vi "DAQmx.Create Trigger.vi"(8 "error in (no error)":errorcluster, 11 "DAQmx in":refnum<class "DAQmx.lvclass">) -> (0 "error out":errorcluster, 3 "DAQmx out":refnum<class "DAQmx.lvclass">)   [LabVIEW 2019, in "DAQmx.lvclass"]
uses:
  DAQmx.lvclass
  typedefs/DAQ.Config.Device Type--enum.ctl
  DAQmx.lvclass/DAQmx.ctl
  a451efbf-a4cf-4ff4-9d43-e4341e5b5646.vi
  <vilib>/DAQmx/configure/trigger.llb/DAQmx Start Trigger (Digital Edge).vi
  <resource>/objmgr/daqmx.rc
panel:
  out "Inventory":cluster{"DAQ Type":T1, "number":i32}[](array[cluster])
  out "DAQ Types":T1[](array[typedef])
  out "SyncPulse.SyncTime 3":dbl[](array[numeric]) format="%#_6p"
  out "SyncPulse.SyncTime 2":dbl[](array[numeric]) format="%#_6p"
  out "master tasks":i32
  out "SyncPulse.SyncTime":dbl format="%#_6p"
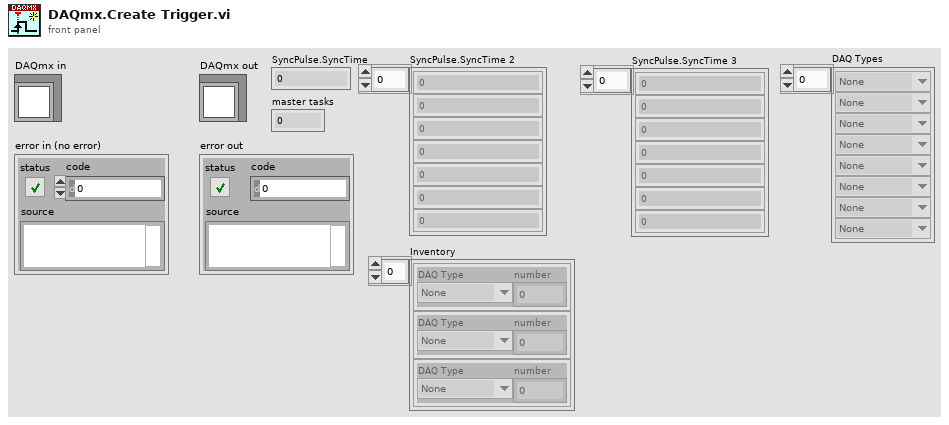
[diagram p1: front panel]
types:
  T1 = typedef "DAQmx.lvclass/DAQ.Config.Device Type--enum.ctl" = enum16{"None", "USB-4431", "PXI-446x"}
  T2 = cluster{"DAQ Type":T1, "Master Tasks":refnum<k21>[], "RefClk.Src":tag, "SyncPulse.Src":tag, "Trigger.Src":tag, "SyncPulse.SyncTime":dbl}
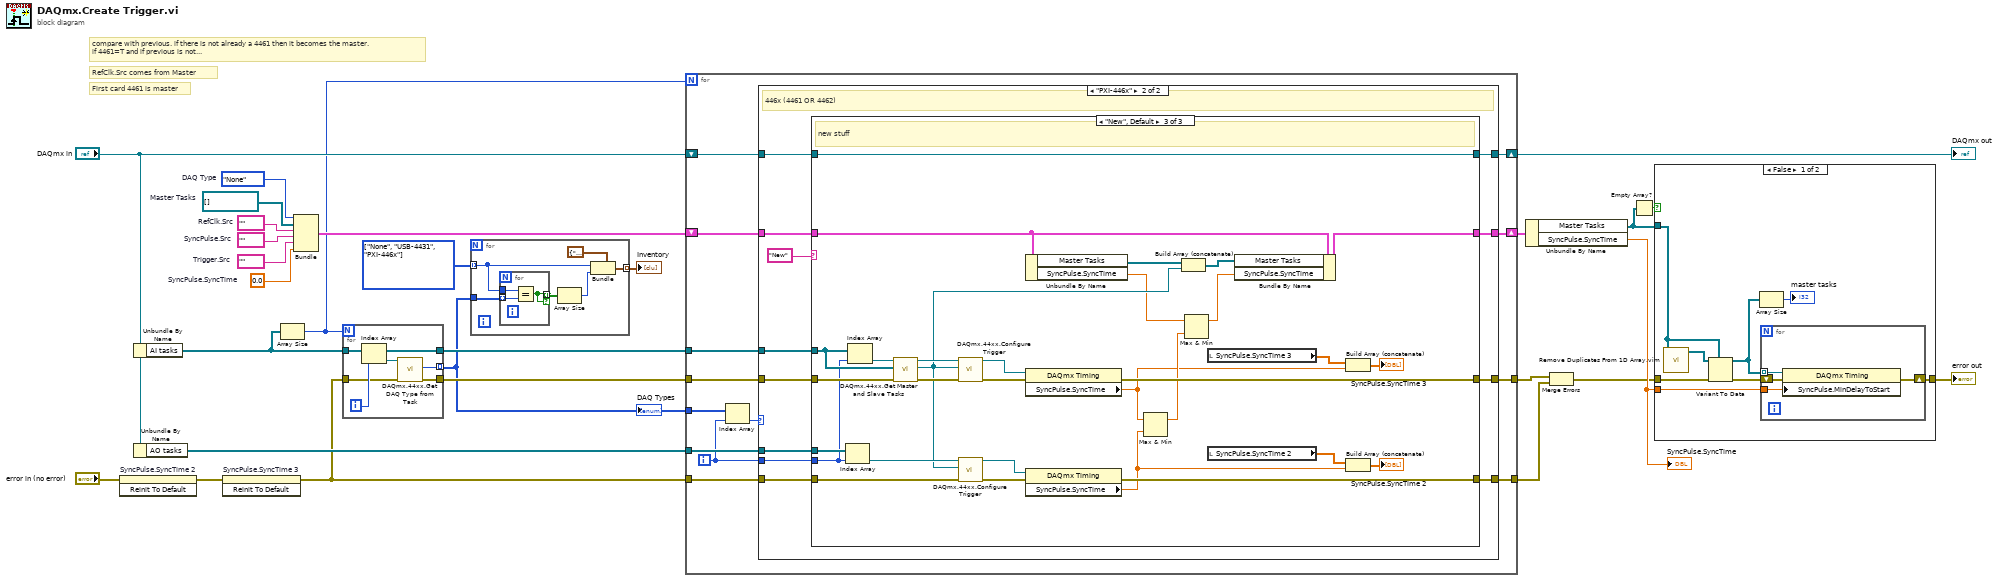
[diagram p0: block diagram]
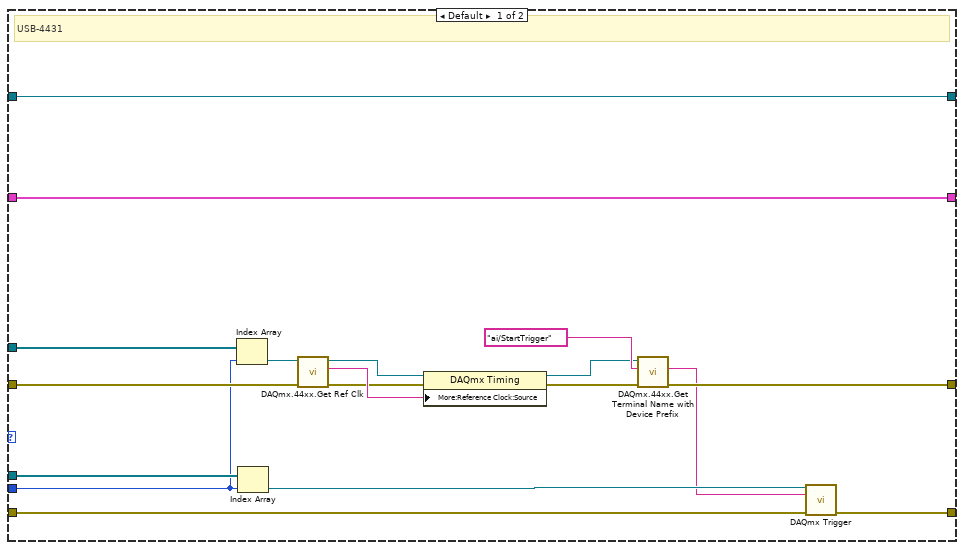
[diagram p2: hidden frame]
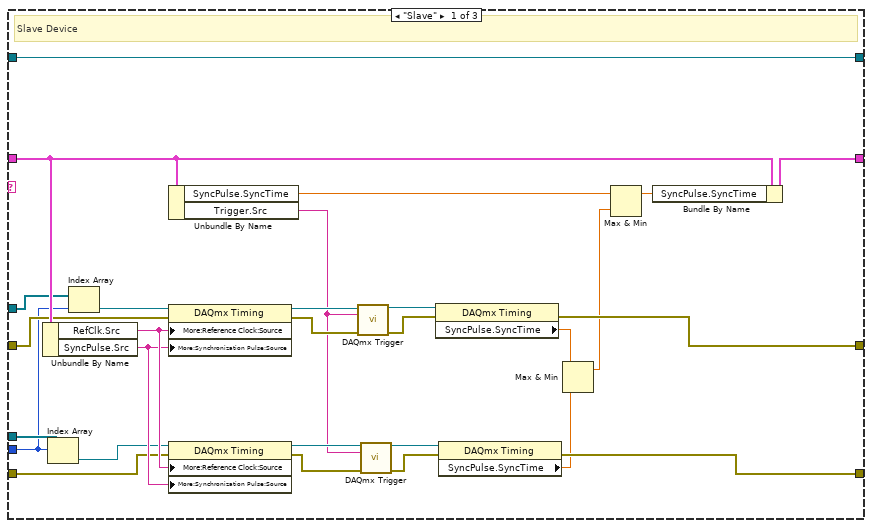
[diagram p3: hidden frame]
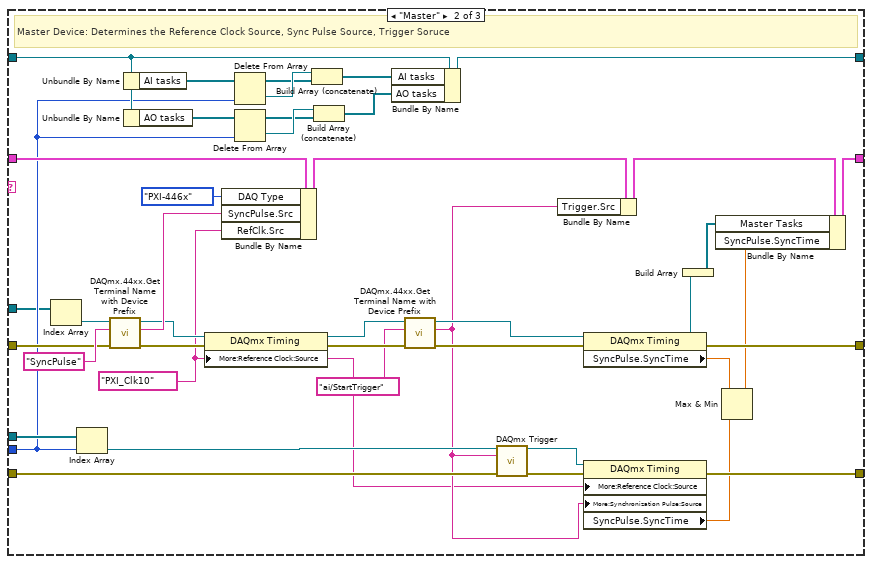
[diagram p4: hidden frame]
diagram:
  w8 = T1[] [enum."None", enum."USB-4431", enum."PXI-446x"] items=["None", "USB-4431", "PXI-446x"] ("y")
  w18 = refnum<k21>[] []  # Master Tasks
  w25 = 0.0  # SyncPulse.SyncTime
  w24 = tag ""  # Trigger.Src
  w23 = tag ""  # SyncPulse.Src
  w20 = tag ""  # RefClk.Src
  w19 = DAQ.Config.Device_Type--enum."None"  # DAQ Type
  # "RefClk.Src comes from Master"
  # "compare with previous. if there is not already a 4461 then it becomes the master. \nif 4461=T and if previous is not..."
  # "First card 4461 is master"
  n1 = invoke on="SyncPulse.SyncTime 2" class="Arr (strict)" method="Reinit To Default"(error in="error in (no error)") -> (error out=w14:errorcluster)  [unwired: 2 in, 2 out]
  n2 = Unbundle By Name("DAQmx in") -> ("AI tasks"=w11:refnum<k21>[])
  n3 = Unbundle By Name("DAQmx in") -> ("AO tasks"=w15:refnum<k21>[])
  n4 = invoke on="SyncPulse.SyncTime 3" class="Arr (strict)" method="Reinit To Default"(error in=w14) -> (error out=w6:errorcluster)  [unwired: 2 in, 2 out]
  n5 = Array Size(array=w11) -> (size(s)=w12:i32)
  n6 = Bundle("DAQ Type"=w19, "Master Tasks"=w18, "RefClk.Src"=w20, "SyncPulse.Src"=w23, "Trigger.Src"=w24, "SyncPulse.SyncTime"=w25) -> (w22:T2)  [unwired: 1 in]
  n7 = for {
    N: w12 -> [_]
    tunnel: w11 -> [w30]
    tunnel: w6 -> [w32]
    tunnel: [w31] -> w10
    tunnel: [w30] -> w9
    tunnel: [w29] -> w7 mode=indexing
    i -> [w34]
    n8 = Index Array(array=w30, index=w34) -> (element=w33:refnum<k21>)
    n9 = call "DAQmx.44xx.Get DAQ Type from Task.vi"("error in (no error)"=w32, "Task in"=w33) -> ("error out"=w31:errorcluster, "DAQ Type"=w29:T1)  [unwired: 5 in, 3 out]
  }
  "DAQ Types" <- w7
  n10 = for {
    tunnel: w7 -> [w39]
    tunnel: w8 -> [w37] mode=indexing
    tunnel: [w36] -> w5 mode=indexing
    n11 = for {
      tunnel: [w43] -> w40 mode=indexing if=w43
      tunnel: w39 -> [w42] mode=indexing
      tunnel: w37 -> [w41]
      n12 = Equal?(x=w41, y=w42) -> (x = y?=w43:bool)
    }
    n13 = Array Size(array=w40) -> (size(s)=w38:i32)
    n14 = Bundle(cluster=cluster{"DAQ Type":T1, "number":i32} {"DAQ Type"=enum."None", "number"=0}, "DAQ Type"=w37, "number"=w38) -> (w36:cluster{"DAQ Type":T1, "number":i32})
  }
  "Inventory" <- w5
  n15 = for {
    N: w12 -> [_]
    tunnel: w9 -> [w48]
    tunnel: w10 -> [w46]
    shift-right: [w55] -> w26
    shift-left: w22 -> [w56]
    tunnel: [w54] -> w4
    tunnel: [w51] -> w2
    tunnel: w6 -> [w50]
    tunnel: w15 -> [w49]
    tunnel: w7 -> [w47]
    shift-right: [w52] -> w21
    shift-left: "DAQmx in" -> [w53]
    i -> [w44]
    n16 = Index Array(array=w47, index=w44) -> (element=w45:T1)
    n17 = case shown="\"PXI-446x\"" w45 {
      tunnel: w56 -> [w74 w86]
      tunnel: [w74 w85] -> w55
      tunnel: w46 -> [w62 w84]
      tunnel: [w66 w83] -> w54
      tunnel: w53 -> [w73 w82]
      tunnel: [w73 w81] -> w52
      tunnel: [w67 w78] -> w51
      tunnel: w50 -> [w68 w80]
      tunnel: w49 -> [w69 w79]
      tunnel: w44 -> [w59 w77]
      tunnel: w48 -> [w60 w76]
      frame Default {
        # "USB-4431"
        n18 = Index Array(array=w60, index=w59) -> (element=w58:refnum<k21>)
        n19 = Index Array(array=w69, index=w59) -> (element=w65:refnum<k21>)
        n20 = call "DAQmx.44xx.Get Ref Clk.vi"("error in (no error)"=w62, "Refnum in"=w58) -> ("error out"=w61:errorcluster, "RefClk.Src"=w64:tag, "Refnum out"=w63:refnum<k21>)  [unwired: 7 in]
        n21 = property class="DAQmx Timing"(reference=w63, error in=w61, "More:Reference Clock:Source"=w64) -> (reference out=w71:refnum<k21>, error out=w70:errorcluster)
        n22 = call "DAQmx.44xx.Get Terminal Name with Device Prefix.vi"("error in (no error)"=w70, "Local Terminal Name"="ai/StartTrigger", "task"=w71) -> ("error out"=w66:errorcluster, "Terminal Name with Device Prefix"=w57:tag)  [unwired: 6 in, 1 out]
        n23 = call-poly <vilib>:"DAQmx Trigger.vi"("task/channels in"=w65, "source"=w57, "error in"=w68) -> ("error out"=w67:errorcluster)  [unwired: 11 in, 1 out]
      }
      frame "PXI-446x" {
        # "446x (4461 OR 4462)"
        n24 = case shown="\"New\", Default" "New" {
          tunnel: w86 -> [w112 w156 w171]
          tunnel: [w111 w145 w172] -> w85
          tunnel: w84 -> [w99 w153 w181]
          tunnel: [w109 w144 w185] -> w83
          tunnel: w82 -> [w108 w134 w183]
          tunnel: [w108 w136 w183] -> w81
          tunnel: w80 -> [w92 w126 w179]
          tunnel: w79 -> [w91 w123 w182]
          tunnel: [w98 w135 w184] -> w78
          tunnel: w77 -> [w88 w122 w160]
          tunnel: w76 -> [w89 w117 w161]
          frame "Slave" {
            # "Slave Device"
            n25 = Unbundle By Name(w112) -> ("RefClk.Src"=w107:tag, "SyncPulse.Src"=w106:tag)
            n26 = Index Array(array=w91, index=w88) -> (element=w90:refnum<k21>)
            n27 = Index Array(array=w89, index=w88) -> (element=w87:refnum<k21>)
            n28 = Unbundle By Name(w112) -> ("SyncPulse.SyncTime"=w95:dbl, "Trigger.Src"=w102:tag)
            n29 = property class="DAQmx Timing"(reference=w87, error in=w99, "More:Reference Clock:Source"=w107, "More:Synchronization Pulse:Source"=w106) -> (reference out=w114:refnum<k21>, error out=w103:errorcluster)
            n30 = property class="DAQmx Timing"(reference=w90, error in=w92, "More:Reference Clock:Source"=w107, "More:Synchronization Pulse:Source"=w106) -> (reference out=w104:refnum<k21>, error out=w101:errorcluster)
            n31 = call-poly <vilib>:"DAQmx Trigger.vi"("task/channels in"=w114, "source"=w102, "error in"=w103) -> ("task out"=w113:refnum<k21>, "error out"=w110:errorcluster)  [unwired: 11 in]
            n32 = call-poly <vilib>:"DAQmx Trigger.vi"("task/channels in"=w104, "source"=w102, "error in"=w101) -> ("task out"=w105:refnum<k21>, "error out"=w100:errorcluster)  [unwired: 11 in]
            n33 = property class="DAQmx Timing"(reference=w113, error in=w110) -> (error out=w109:errorcluster, "SyncPulse.SyncTime"=w93:dbl)  [unwired: 1 out]
            n34 = property class="DAQmx Timing"(reference=w105, error in=w100) -> (error out=w98:errorcluster, "SyncPulse.SyncTime"=w97:dbl)  [unwired: 1 out]
            n35 = Max & Min(x=w93, y=w97) -> (max(x,y)=w96:dbl)  [unwired: 1 out]
            n36 = Max & Min(x=w95, y=w96) -> (max(x,y)=w94:dbl)  [unwired: 1 out]
            n37 = Bundle By Name(cluster=w112, "SyncPulse.SyncTime"=w94) -> (w111:T2)
          }
          frame "Master" {
            w115 = tag "PXI_Clk10" ("RefClk.Src")
            # "Master Device: Determines the Reference Clock Source, Sync Pulse Source, Trigger Soruce"
            n38 = Index Array(array=w117) -> (element=w120:refnum<k21>)  [unwired: 1 in]
            n39 = Index Array(array=w123, index=w122) -> (element=w121:refnum<k21>)
            n40 = call "DAQmx.44xx.Get Terminal Name with Device Prefix.vi"("error in (no error)"=w153, "Local Terminal Name"="SyncPulse", "task"=w120) -> ("error out"=w152:errorcluster, "Terminal Name with Device Prefix"=w154:tag, "task out"=w142:refnum<k21>)  [unwired: 6 in]
            n41 = Unbundle By Name(w134) -> ("AI tasks"=w140:refnum<k21>[])
            n42 = Unbundle By Name(w134) -> ("AO tasks"=w133:refnum<k21>[])
            n43 = property class="DAQmx Timing"(reference=w142, error in=w152, "More:Reference Clock:Source"=w115) -> (reference out=w149:refnum<k21>, error out=w151:errorcluster)
            n44 = Bundle By Name(cluster=w156, "DAQ Type"=DAQ.Config.Device_Type--enum."PXI-446x", "SyncPulse.Src"=w154, "RefClk.Src"=w115) -> (w148:T2)
            n45 = Delete From Array(array=w140, index=w122) -> (deleted portion=w139:refnum<k21>, array with subset deleted=w138:refnum<k21>[])  [unwired: 1 in]
            n46 = Delete From Array(array=w133, index=w122) -> (deleted portion=w132:refnum<k21>, array with subset deleted=w131:refnum<k21>[])  [unwired: 1 in]
            n47 = Build Array (concatenate)(w139, w138) -> (w137:refnum<k21>[])
            n48 = Build Array (concatenate)(w132, w131) -> (w130:refnum<k21>[])
            n49 = Bundle By Name(cluster=w134, "AI tasks"=w137, "AO tasks"=w130) -> (w136:refnum<class "DAQmx.lvclass">)
            n50 = call "DAQmx.44xx.Get Terminal Name with Device Prefix.vi"("error in (no error)"=w151, "Local Terminal Name"="ai/StartTrigger", "task"=w149) -> ("error out"=w146:errorcluster, "Terminal Name with Device Prefix"=w116:tag, "task out"=w147:refnum<k21>)  [unwired: 6 in]
            n51 = call-poly <vilib>:"DAQmx Trigger.vi"("task/channels in"=w121, "source"=w116, "error in"=w126) -> ("task out"=w124:refnum<k21>, "error out"=w125:errorcluster)  [unwired: 11 in]
            n52 = Bundle By Name(cluster=w148, "Trigger.Src"=w116) -> (w143:T2)
            n53 = property class="DAQmx Timing"(reference=w147, error in=w146) -> (reference out=w141:refnum<k21>, error out=w144:errorcluster, "SyncPulse.SyncTime"=w129:dbl)
            n54 = property class="DAQmx Timing"(reference=w124, error in=w125, "More:Reference Clock:Source"=w115, "More:Synchronization Pulse:Source"=w116) -> (error out=w135:errorcluster, "SyncPulse.SyncTime"=w128:dbl)  [unwired: 1 out]
            n55 = Build Array(w141) -> (w118:refnum<k21>[])
            n56 = Max & Min(x=w129, y=w128) -> (max(x,y)=w127:dbl)  [unwired: 1 out]
            n57 = Bundle By Name(cluster=w143, "Master Tasks"=w118, "SyncPulse.SyncTime"=w127) -> (w145:T2)
          }
          frame "New", Default {
            # "new stuff"
            n58 = Index Array(array=w182, index=w160) -> (element=w177:refnum<k21>)
            n59 = Index Array(array=w161, index=w160) -> (element=w173:refnum<k21>)
            n60 = call "DAQmx.44xx.Get Master and Slave Tasks.vi"("error in (no error)"=w181, "AI tasks in"=w161, "AI task"=w173) -> ("error out"=w180:errorcluster, "master task"=w166:refnum<k21>, "AI task out"=w178:refnum<k21>)  [unwired: 6 in]
            n61 = call "DAQmx.44xx.Configure Trigger.vi"("error in (no error)"=w180, "master task in"=w166, "task in"=w178) -> ("error out"=w186:errorcluster, "task out"=w176:refnum<k21>)  [unwired: 7 in]
            n62 = call "DAQmx.44xx.Configure Trigger.vi"("error in (no error)"=w179, "master task in"=w166, "task in"=w177) -> ("error out"=w174:errorcluster, "task out"=w175:refnum<k21>)  [unwired: 7 in]
            n63 = Unbundle By Name(w171) -> ("Master Tasks"=w168:refnum<k21>[], "SyncPulse.SyncTime"=w157:dbl)
            n64 = property class="DAQmx Timing"(reference=w176, error in=w186) -> (error out=w185:errorcluster, "SyncPulse.SyncTime"=w162:dbl)  [unwired: 1 out]
            n65 = property class="DAQmx Timing"(reference=w175, error in=w174) -> (error out=w184:errorcluster, "SyncPulse.SyncTime"=w165:dbl)  [unwired: 1 out]
            n66 = Max & Min(x=w162, y=w165) -> (max(x,y)=w170:dbl)  [unwired: 1 out]
            n67 = Build Array (concatenate)(w168, w166) -> (w167:refnum<k21>[])
            n68 = Max & Min(x=w157, y=w170) -> (max(x,y)=w169:dbl)  [unwired: 1 out]
            n69 = local read "SyncPulse.SyncTime 3"() -> (w158:dbl[])
            n70 = local read "SyncPulse.SyncTime 2"() -> (w159:dbl[])
            n71 = Bundle By Name(cluster=w171, "Master Tasks"=w167, "SyncPulse.SyncTime"=w169) -> (w172:T2)
            n72 = Build Array (concatenate)(w158, w162) -> (→"SyncPulse.SyncTime 3":dbl[])
            n73 = Build Array (concatenate)(w159, w165) -> (→"SyncPulse.SyncTime 2":dbl[])
          }
        }
      }
    }
  }
  "DAQmx out" <- w21
  n74 = Unbundle By Name(w26) -> ("Master Tasks"=w1:refnum<k21>[], "SyncPulse.SyncTime"=w17:dbl)
  "SyncPulse.SyncTime" <- w17
  n75 = Merge Errors(w4, w2) -> (w3:errorcluster)
  n76 = Empty Array?(array=w1) -> (empty?=w27:bool)
  n77 = case shown="False" w27 {
    tunnel: w1 -> [w189 _]
    tunnel: w17 -> [w194 _]
    tunnel: w3 -> [w191 w199]
    tunnel: [w193 w199] -> w28
    frame False {
      n78 = call "Remove Duplicates From 1D Array.vim"("array"=w189) -> ("array with duplicates removed"=w192:refnum<k21>[])  [unwired: 10 in]
      n79 = Variant To Data(error in=w191, type=w189, Variant=w192) -> (data=w187:refnum<k21>[], error out=w190:errorcluster)
      n80 = Array Size(array=w187) -> (size(s)=→"master tasks":i32)
      n81 = for {
        tunnel: w194 -> [w198]
        shift-right: [w196] -> w193
        shift-left: w190 -> [w197]
        tunnel: w187 -> [w195] mode=indexing
        n82 = property class="DAQmx Timing"(reference=w195, error in=w197, "SyncPulse.MinDelayToStart"=w198) -> (error out=w196:errorcluster)  [unwired: 1 out]
      }
    }
    frame True {
      # "If master task=empty, then no master devices were ever found (ie, all 4431s)"
    }
  }
  "error out" <- w28
